vi "To Generic.vi"(8 "error in (no error)":errorcluster, 11 "Instrument Error Data in":refnum<class "DMM Measurement Data.lvclass">) -> (0 "error out":errorcluster, 2 "Generic Data":refnum<class "Generic Data.lvclass">[](array[class]), 3 "Data Name":string[](array[string]))   [LabVIEW 2020, in "DMM Msg.lvlib" / "DMM Measurement Data.lvclass"]
doc: "Present private data as an array of named generic data elements."
uses:
  DMM Measurement Data.lvclass
  PPL/HDH.Data.Generic.lvlibp/Generic Data/Generic Data.lvclass
  DMM Measurement Data.lvclass/DMM Measurement Data.ctl
  PPL/HDH.Data.Generic.lvlibp/Generic Data/Boolean/Boolean.lvclass
  C:/Current projects/WS/PPL/HDH.Data.Generic.lvlibp/Generic Data/Generic Data.lvclass
  PPL/HDH.Data.Generic.lvlibp/Generic Data/Double/Double.lvclass
  PPL/HDH.Data.Generic.lvlibp/Generic Data/I32/I32.lvclass
  PPL/HDH.Data.Generic.lvlibp/Generic Data/U32/U32.lvclass
  PPL/HDH.Data.Generic.lvlibp/Generic Data/String/String.lvclass
  PPL/HDH.Data.Generic.lvlibp/Generic Data/Generic Array Data/Double Array/Double Array.lvclass
  PPL/HDH.Actor Framework.Core.Instrument Handler.lvlibp/Data/Instrument Data/Instrument Data.lvclass
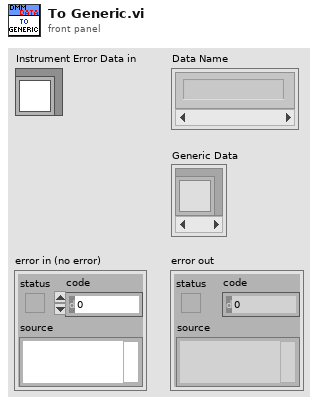
[diagram p1: front panel]
types:
  T1 = typedef "HDH.Driver.DMM.lvlibp/Ctl_Function.ctl" = enum8{"DC Volts", "AC Volts", "DC Current", "AC Current", "2-wire Resistance", "4-wire Resistance", "Diode", "Frequency", "Period", "AC Volts DC Coupled", "Capacitance", "Inductance", "Temperature"}
  T2 = typedef "HDH.Driver.DMM.lvlibp/Ctl_DigitResolution.ctl" = enum8{"3½", "4½", "5½", "6½", "7½"}
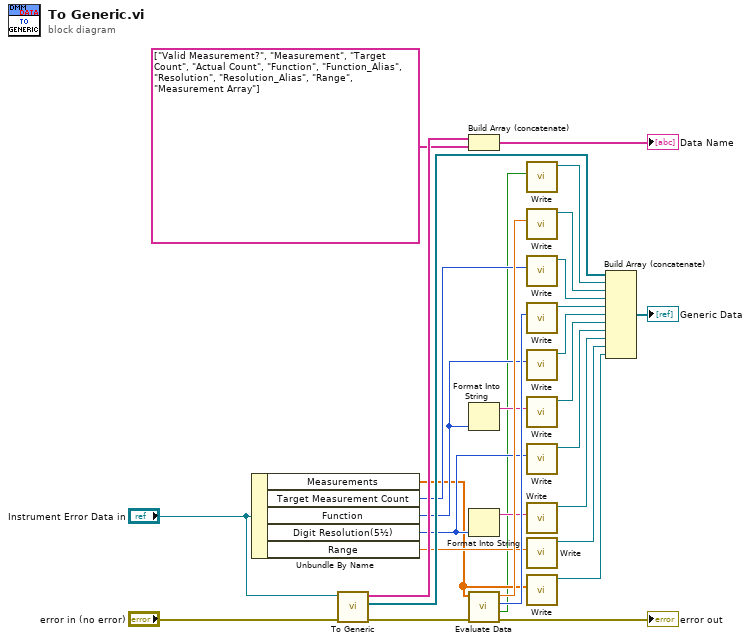
[diagram p0: block diagram]
diagram:
  n1 = Unbundle By Name("Instrument Error Data in") -> ("Measurements"=w4:dbl[], "Target Measurement Count"=w18:i32, "Function"=w13:T1, "Digit Resolution(5½)"=w9:T2, "Range"=w6:dbl)
  n2 = call-parent "To Generic.vi"("error in (no error)"="error in (no error)", "Instrument Error Data in"="Instrument Error Data in") -> ("error out"=w26:errorcluster, "Generic Data"=w23:refnum<class "Generic Data.lvclass">[], "Data Name"=w29:string[])  [unwired: 7 in]
  n3 = Build Array (concatenate)(w29, string[] ["Valid Measurement?", "Measurement", "Target Count", "Actual Count", "Function", "Function_Alias", "Resolution", "Resolution_Alias", "Range", "Measurement Array"] ("Data Name")) -> (→"Data Name":string[])
  n4 = Format Into String(w13) -> (resulting string=w12:string)  [unwired: 3 in, 1 out]
  n5 = Format Into String(w9) -> (resulting string=w10:string)  [unwired: 3 in, 1 out]
  n6 = call "Evaluate Data.vi"("error in (no error)"=w26, "Measurements"=w4) -> ("error out"=→"error out":errorcluster, "Valid Data?"=w2:bool, "Measurement Count"=w16:i32, "Average"=w24:dbl)  [unwired: 6 in]
  n7 = call "Write.vi"("Boolean"=w2) -> ("Boolean out"=w1:refnum<class "Boolean.lvclass">)  [unwired: 10 in]
  n8 = call "Write.vi"("Double"=w24) -> ("Double out"=w19:refnum<class "Double.lvclass">)  [unwired: 10 in]
  n9 = call "Write.vi"("I32"=w18) -> ("I32 out"=w17:refnum<class "I32.lvclass">)  [unwired: 10 in]
  n10 = call "Write.vi"("I32"=w16) -> ("I32 out"=w15:refnum<class "I32.lvclass">)  [unwired: 10 in]
  n11 = call "Write.vi"("U32"=w13) -> ("U32 out"=w14:refnum<class "U32.lvclass">)  [unwired: 10 in]
  n12 = call "Write.vi"("String"=w12) -> ("String out"=w11:refnum<class "String.lvclass">)  [unwired: 10 in]
  n13 = call "Write.vi"("U32"=w9) -> ("U32 out"=w8:refnum<class "U32.lvclass">)  [unwired: 10 in]
  n14 = call "Write.vi"("String"=w10) -> ("String out"=w7:refnum<class "String.lvclass">)  [unwired: 10 in]
  n15 = call "Write.vi"("Double"=w6) -> ("Double out"=w5:refnum<class "Double.lvclass">)  [unwired: 10 in]
  n16 = call "Write.vi"("Double Array"=w4) -> ("Double Array out"=w3:refnum<class "Double Array.lvclass">)  [unwired: 10 in]
  n17 = Build Array (concatenate)(w23, w1, w19, w17, w15, w14, w11, w8, w7, w5, w3) -> (→"Generic Data":refnum<class "Generic Data.lvclass">[])
